vi "Generate Unique IDs Priv.vi"(8 "Error In":errorcluster, 10 "# IDs (1)":i32=1, 11 "Tree Dictionary":variant) -> (0 "Error Out":errorcluster, 1 "IDs":string[](array[string]), 2 "First ID":string, 3 "Tree Dictionary Out":variant)   [LabVIEW 2017, in "Tree API.lvlib" / "Tree.lvclass"]
uses:
  Tree.lvclass
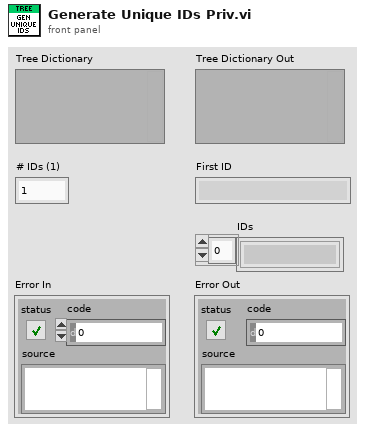
[diagram p1: front panel]
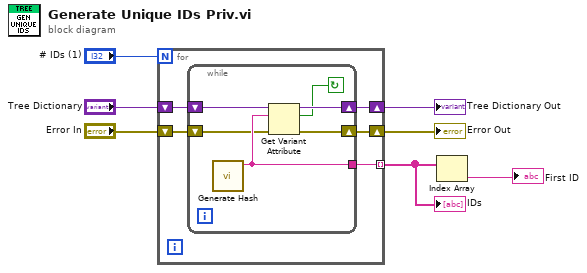
[diagram p0: block diagram]
diagram:
  n1 = for {
    N: "# IDs (1)" -> [_]
    shift-right: [w11] -> w5
    shift-left: "Tree Dictionary" -> [w12]
    tunnel: [w10] -> w2 mode=indexing
    shift-right: [w8] -> w7
    shift-left: "Error In" -> [w9]
    n2 = while {
      shift-right: [w17] -> w11
      shift-left: w12 -> [w18]
      tunnel: [w15] -> w10
      shift-right: [w13] -> w8
      shift-left: w9 -> [w14]
      stop <- w16 continue-if-true
      n3 = call "Generate Hash.vi"() -> ("Hash"=w15:string)  [unwired: 10 in, 1 out]
      n4 = Get Variant Attribute(Variant=w18, name=w15, error in=w14) -> (duplicate Variant=w17:variant, found=w16:bool, error out=w13:errorcluster)  [unwired: 1 in, 1 out]
    }
  }
  "Error Out" <- w7
  "Tree Dictionary Out" <- w5
  "IDs" <- w2
  n5 = Index Array(array=w2) -> (element=→"First ID":string)  [unwired: 1 in]
